vi "Save Data.vi"(8 "error in (no error)":errorcluster, 10 "Temp File Array":T1(array[cluster]), 11 "refnum in":refnum<file>) -> (0 "error out":errorcluster, 2 "Section offset":i32, 3 "refnum out":refnum<file>)   [LabVIEW 2009]
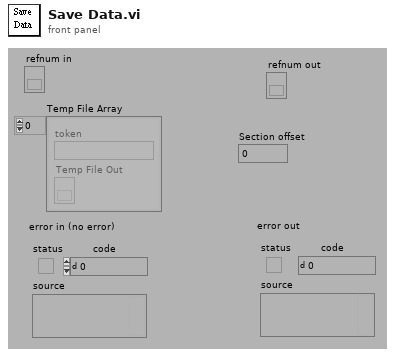
[diagram p1: front panel]
types:
  T1 = cluster{"token":string, "Temp File Out":refnum<file>}[]
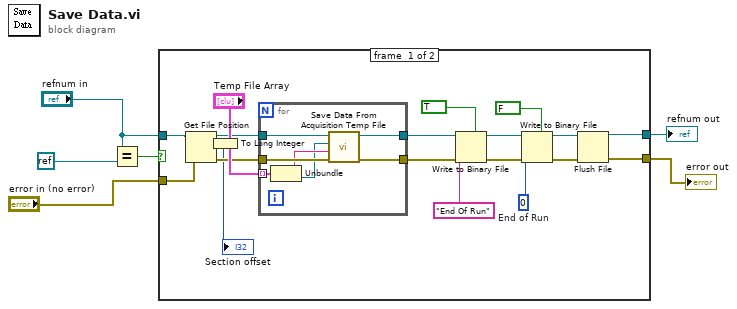
[diagram p0: block diagram]
diagram:
  n1 = Equal?(x="refnum in", y=refnum<k0> refnum) -> (x = y?=w1:bool)
  n2 = case shown="False" w1 {
    tunnel: "error in (no error)" -> [w11 w34]
    tunnel: [w18 w34] -> w6
    tunnel: "refnum in" -> [w13 w33]
    tunnel: [w17 w33] -> w5
    frame #0 {
      w25 = 0  # End of Run
      n3 = Get File Position(4:w11, 7:w13) -> (0:w10:errorcluster, 2:w8:i64, 3:w12:refnum<file>)
      n4 = To Long Integer(number=w8) -> (32bit integer=→"Section offset":i32)
      n5 = for {
        tunnel: w10 -> [w32]
        tunnel: w12 -> [w31]
        tunnel: [w30] -> w16
        tunnel: [w29] -> w15
        tunnel: "Temp File Array" -> [w28] mode=indexing
        n6 = Unbundle(w28) -> ("token"=w27:string, "Temp File Out"=w26:refnum<file>)
        n7 = call "Save Data From Acquisition Temp File.vi"("error in"=w32, "Type"=w27, "Arrival Time Temp File"=w26, "refnum in"=w31) -> ("error out"=w29:errorcluster, "refnum"=w30:refnum<file>)  [unwired: 6 in]
      }
      n8 = Write to Binary File(file (use dialog)=w16, data="End Of Run", error in=w15, 5:TRUE ("header (F)")) -> (refnum out=w24:refnum<file>, error out=w23:errorcluster)  [unwired: 2 in, 1 out]
      n9 = Write to Binary File(file (use dialog)=w24, data=w25, error in=w23, 5:FALSE ("prepend array or string size? (T)")) -> (refnum out=w20:refnum<file>, error out=w19:errorcluster)  [unwired: 2 in, 1 out]
      n10 = Flush File(refnum=w20, error in=w19) -> (refnum out=w17:refnum<file>, error out=w18:errorcluster)
    }
    frame #1 {
    }
  }
  "error out" <- w6
  "refnum out" <- w5
